vi "Save Data.vi"(8 "error in (no error)":errorcluster, 11 "Tektronix Driver in":refnum<class "Tektronix Driver.lvclass">) -> (0 "error out":errorcluster, 1 "Finished":bool, 2 "Current read position":i32, 3 "Tektronix Driver out":refnum<class "Tektronix Driver.lvclass">)   [LabVIEW 2020, in "Tektronix Driver.lvclass"]
uses:
  Tektronix Driver.lvclass
  C:/GitHub/NHMFL_Core/Libraries/Instruments/Pulse Driver/Pulse Driver.lvclass
  C:/GitHub/NHMFL_Core/Libraries/Instruments/Instrument Driver/Instrument Driver.lvclass
  Pulse Driver/Pulse Driver.lvclass/Pulse Driver.ctl
  Pulse Driver/Read tdms file.vi
  Pulse Driver/Write tdms file.vi
  <vilib>/Waveform/WDTOps.llb/WDT Number of Waveform Samples DBL.vi
  <instrlib>/Tektronix 7000 Series/Tektronix 7000 Series.lvlib
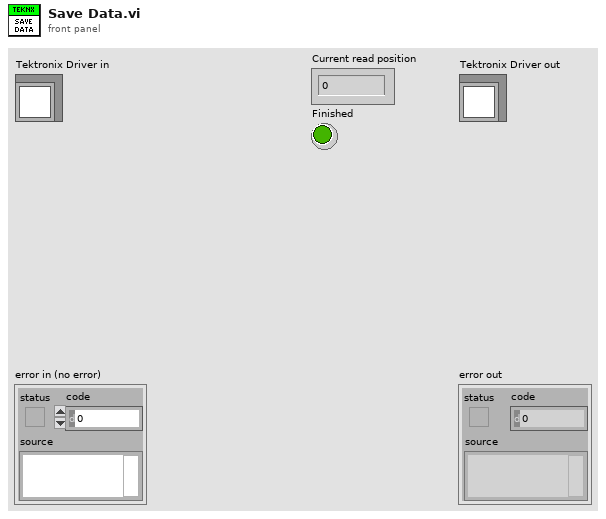
[diagram p1: front panel]
types:
  T1 = typedef "Tektronix Configuration.ctl" = cluster{"Channel":i32, "Number of averages":i32, "Input impedace":enum16{"1 M Ohm", "50 Ohm"}, "Vertical coupling":enum16{"AC", "DC", "Ground"}}
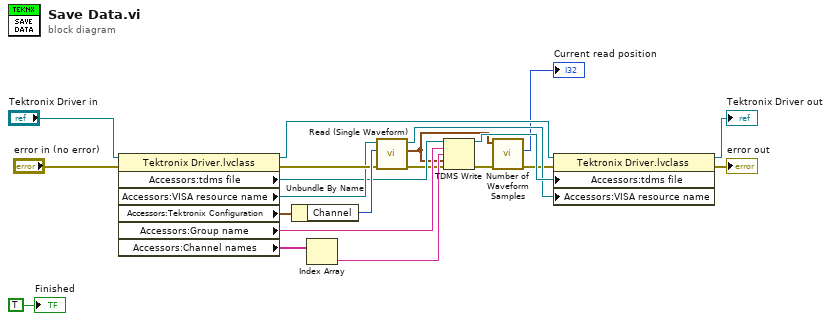
[diagram p0: block diagram]
diagram:
  n1 = property class="Tektronix Driver.lvclass"(reference="Tektronix Driver in", error in="error in (no error)") -> (reference out=w11:refnum<class "Tektronix Driver.lvclass">, error out=w17:errorcluster, "Accessors:tdms file"=w15:refnum<k34>, "Accessors:VISA resource name"=w16:refnum<visa-resource-name>, "Accessors:Tektronix Configuration"=w19:T1, "Accessors:Group name"=w14:string, "Accessors:Channel names"=w13:string[])
  n2 = Unbundle By Name(w19) -> ("Channel"=w18:i32)
  n3 = Index Array(array=w13) -> (element=w12:string)  [unwired: 1 in]
  n4 = call <instrlib>:"Read (Single Waveform).vi"("error in (no error)"=w17, "Channel (0: Channel 1)"=w18, "VISA resource name"=w16) -> ("error out"=w8:errorcluster, "Waveform Data"=w4:waveform(dbl), "VISA resource name out"=w9:refnum<visa-resource-name>)  [unwired: 6 in]
  n5 = TDMS Write(0:w15, 5:w14, 7:w12, 9:w4, 11:w8) -> (4:w10:refnum<k34>, 15:w3:errorcluster)  [unwired: 1 in, 2 out]
  n6 = call-poly <vilib>:"Number of Waveform Samples.vi"("error in (no error)"=w3, "waveform in"=w4) -> ("error out"=w2:errorcluster, "number of samples"=→"Current read position":i32)  [unwired: 7 in, 1 out]
  n7 = property class="Tektronix Driver.lvclass"(reference=w11, error in=w2, "Accessors:tdms file"=w10, "Accessors:VISA resource name"=w9) -> (reference out=→"Tektronix Driver out":refnum<class "Tektronix Driver.lvclass">, error out=→"error out":errorcluster)
  "Finished" <- TRUE ("Finished")
